vi "Configure Current Limit.vi"(8 "error in (no error)":errorcluster, 10 "Current Limit Setting":cluster{"Address":dbl, "Current Limit":dbl}, 11 "BK-Precision in":refnum<class "BK-Precision.lvclass">) -> (0 "error out":errorcluster, 3 "BK-Precision out":refnum<class "BK-Precision.lvclass">)   [LabVIEW 2016, in "DC PWS.lvlib" / "BK-Precision.lvclass"]
uses:
  BK-Precision.lvclass
  BK-Precision.lvclass/BK-Precision.ctl
  <instrlib>/BK Precision 911X Series/BK Precision 911X Series.lvlib
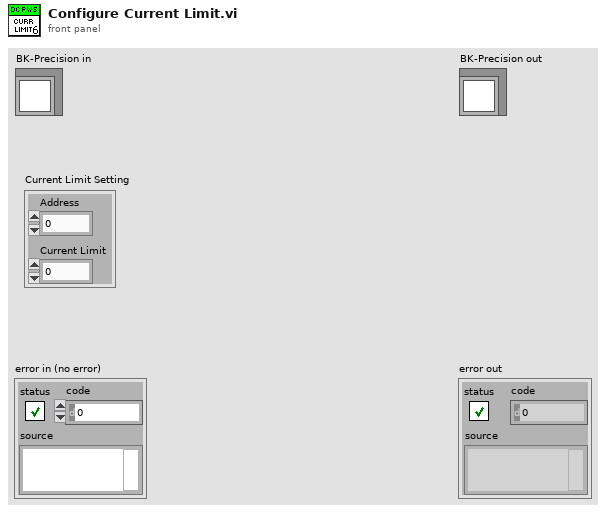
[diagram p1: front panel]
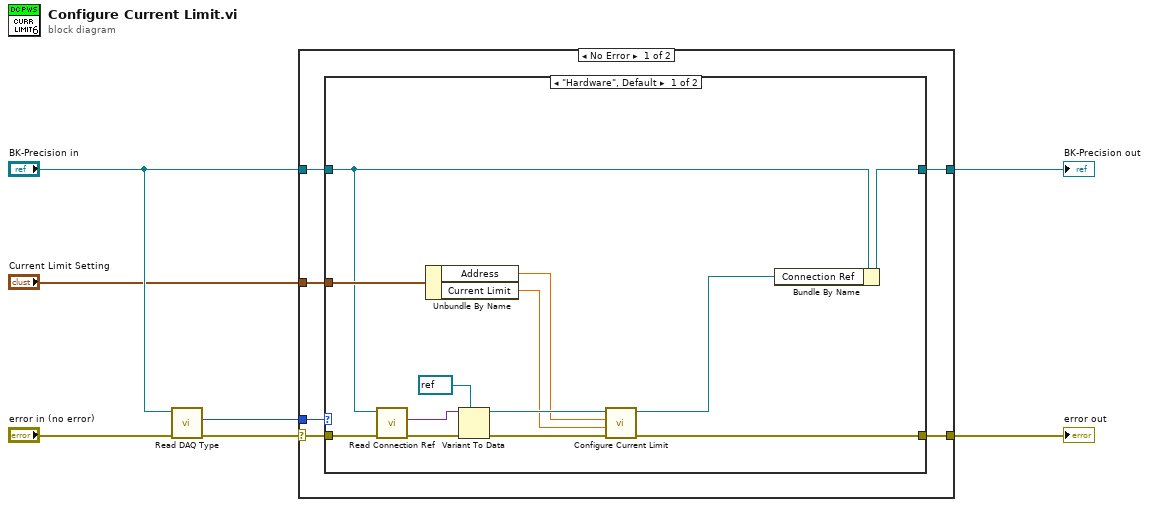
[diagram p0: block diagram]
diagram:
  n1 = call "Read DAQ Type.vi"("error in (no error)"="error in (no error)", "BK-Precision in"="BK-Precision in") -> ("error out"=w6:errorcluster, "Type"=w5:enum16{"Hardware", "Simulation"})  [unwired: 7 in, 1 out]
  n2 = case shown="No Error" w6 {
    selector: w6 -> [w10 w29]
    tunnel: w5 -> [w13 _]
    tunnel: "BK-Precision in" -> [w12 w30]
    tunnel: "Current Limit Setting" -> [w11 _]
    tunnel: [w9 w30] -> w2
    tunnel: [w8 w29] -> w1
    frame No Error {
      n3 = case shown="\"Hardware\", Default" w13 {
        tunnel: w12 -> [w17 w28]
        tunnel: w11 -> [w20 _]
        tunnel: w10 -> [w26 w27]
        tunnel: [w16 w28] -> w9
        tunnel: [w14 w27] -> w8
        frame "Hardware", Default {
          n4 = call "Read Connection Ref.vi"("error in (no error)"=w26, "BK-Precision in"=w17) -> ("error out"=w25:errorcluster, "Conn Ref"=w23:variant)  [unwired: 7 in, 1 out]
          n5 = Unbundle By Name(w20) -> ("Address"=w19:dbl, "Current Limit"=w18:dbl)
          n6 = Variant To Data(error in=w25, type=refnum<visa-resource-name> refnum ("VISA resource name"), Variant=w23) -> (data=w21:refnum<visa-resource-name>, error out=w24:errorcluster)
          n7 = call <instrlib>:"Configure Current Limit.vi"("error in (no error)"=w24, "Current Limit (0.0 A)"=w18, "Address (0)"=w19, "VISA resource name"=w21) -> ("error out"=w14:errorcluster, "VISA resource name out"=w15:refnum<visa-resource-name>)  [unwired: 6 in]
          n8 = Bundle By Name(cluster=w17, "Connection Ref"=w15) -> (w16:refnum<class "BK-Precision.lvclass">)
        }
        frame "Simulation" {
        }
      }
    }
    frame Error {
    }
  }
  "error out" <- w1
  "BK-Precision out" <- w2
